vi "读取LoggerQueueRef.vi"(8 "error in (no error)":errorcluster caption="错误输入（无错误）", 11 "Logger输入":refnum<class "Logger.lvclass">) -> (0 "error out":errorcluster caption="错误输出", 2 "LoggerQueueRef":refnum<queue>, 3 "Logger输出":refnum<class "Logger.lvclass">)   [LabVIEW 2019, in "Logger.lvclass"]
uses:
  <userlib>/Logger/Logger.lvclass
  <userlib>/Logger/Ctls/LoggerMessage.ctl
  <userlib>/Logger/Logger.lvclass/Logger.ctl
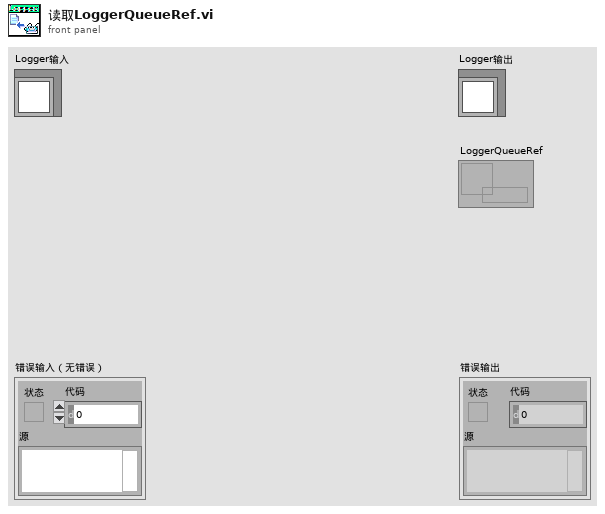
[diagram p1: front panel]
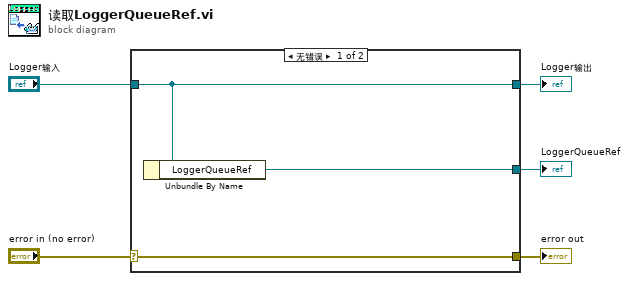
[diagram p0: block diagram]
diagram:
  n1 = case shown="无错误" "error in (no error)" {
    selector: "error in (no error)" -> [w8 w9]
    tunnel: [w8 w9] -> w4
    tunnel: [w7 w10] -> w2
    tunnel: "Logger输入" -> [w7 w10]
    tunnel: [w6 _] -> w1
    frame No Error {
      n2 = Unbundle By Name(w7) -> ("LoggerQueueRef"=w6:refnum<queue>)
    }
    frame Error {
    }
  }
  "error out" <- w4
  "Logger输出" <- w2
  "LoggerQueueRef" <- w1
